vi "AIT 1553 RT Driver VI.vi"(7 "Operation":T1, 11 "Device Reference in":T2 format="%.0x") -> (0 "Error Code":i32)   [LabVIEW 2013, in "AIT 1553 Custom Device.lvlib"]
uses:
  AIT 1553 Custom Device.lvlib
  <vilib>/NI Veristand/Custom Device API/Custom Device Item Ref.ctl
  <vilib>/NI Veristand/Custom Device API/Hardware Interface Driver VI Operation.ctl
  RT Controls/AIT 1553  - RT Data.ctl
  RT Controls/AIT 1553 - RT HW Channel.ctl
  RT Controls/AIT 1553 - Bus Section.ctl
  RT Controls/AIT 1553 - RT Message Settings.ctl
  <vilib>/NI Veristand/Custom Device API/Block Data Reference.ctl
  <vilib>/NI Veristand/Custom Device API/Data Reference.ctl
  RT Controls/AIT 1553 - Driver Data.ctl
  Controls and Global/Start Bit.ctl
  Controls and Global/Number of Bits.ctl
  RT Controls/AIT 1553 - Board Config Info.ctl
  RT Controls/AIT 1553 - Hardware Type.ctl
  RT Controls/Error Qs.ctl
  RT Controls/Status Channels Config.ctl
  RT Controls/FIFO.ctl
  RT Controls/Label Transfer Config.ctl
  <vilib>/NI Veristand/Custom Device Tools/Custom Device Utility Library/RT Debug String Color Spec.ctl
  RT Controls/Async Loop Control Enum.ctl
  RT Controls/ReadWrite Selector.ctl
  SubVIs/Data Ref FGV.vi
  <vilib>/NI Veristand/Custom Device API/NI VeriStand - Set Channel Value by Data Reference.vi
  SubVIs/Error/Push Error if Different.vi
  SubVIs/Error/Print Error.vi
  SubVIs/Init/AIT 1553 - Separate Tx-Rx Messages.vi
  SubVIs/Init/AIT 1553 - Parse RT Channels.vi
  SubVIs/Init/AIT 1553 - Parse BM Channels.vi
  SubVIs/Init/AIT 1553 - Parse BC Channels.vi
  Controls and Global/Global.vi
  SubVIs/Init/AIT 1553 - Get Index and Length.vi
  <vilib>/NI Veristand/Custom Device API/Global Data Refs.vi
  <vilib>/NI Veristand/Custom Device API/Custom Device API.lvlib
  <instrlib>/AIT 1553/AIT 1553.lvlib
  <vilib>/NI Veristand/Custom Device Tools/Custom Device Utility Library/Custom Device Utility Library.lvlib
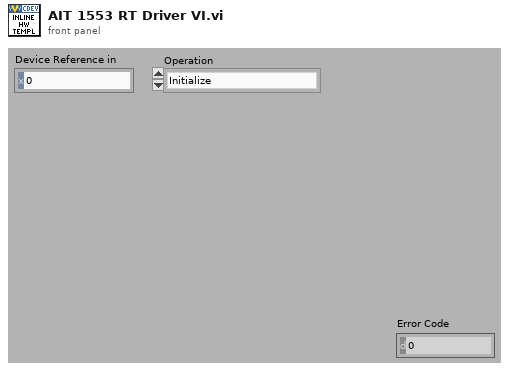
[diagram p1: front panel]
types:
  T1 = typedef "Custom Device API.lvlib/Hardware Interface Driver VI Operation.ctl" = enum16{"Initialize", "Start", "Read Data from HW", "Write Data to HW", "Close"}
  T2 = typedef "Custom Device API.lvlib/Custom Device Item Ref.ctl" = u64
  T3 = typedef "AIT 1553 Custom Device.lvlib/AIT 1553  - RT Data.ctl" = cluster{"HWInput Channels":T4[], "HWOutput Channels":T4[], "Bus Config Info":T12, "Start":refnum<notifier>, "HWIn BaseRate - BC or RT":i64, "HWOut BaseRate - BC or RT":i64, "HWIn BaseRate - BM":i64, "Error Qs":T14, "Error Pub Q":refnum<queue>, "Status Config":T15, "FIFOs":T16, "VI Refs":refnum<vi>[], "Label Transfer Config":T17, "Acyclic Frame Refs":T2[]}
  T4 = typedef "AIT 1553 Custom Device.lvlib/AIT 1553 - RT HW Channel.ctl" = cluster{"channel #":u16, "channel handle":u32, "Bus Section":T5, "Msg Names":string[], "Message Settings":T6[]}
  T5 = typedef "AIT 1553 Custom Device.lvlib/AIT 1553 - Bus Section.ctl" = enum16{"BC", "BM", "RT"}
  T6 = typedef "AIT 1553 Custom Device.lvlib/AIT 1553 - RT Message Settings.ctl" = cluster{"Name":string, "xmlName":string, "Tx-Rx_T-Tx":bool, "RT_Address":u8, "RT_SA_Address":u8, "Block Data Refs":T7[], "Values Array":dbl[], "Length":i32, "Words":i32, "FIFO Index":i32, "RX Word":u32, "transfer handle":u32, "IterationOffset":i32, "Default Msg Data":u16[], "Driver Data":T9, "Status Data":u32[]}
  T7 = typedef "Custom Device API.lvlib/Block Data Reference.ctl" = cluster{"Data Reference":T8, "Offset":i32, "Length":i32}
  T8 = typedef "Custom Device API.lvlib/Data Reference.ctl" = i32
  T9 = typedef "AIT 1553 Custom Device.lvlib/AIT 1553 - Driver Data.ctl" = cluster{"First Word":T10[], "Start Bit":T10[], "Num Bits":T11[], "Decimation":i32, "IterationOffset":i32, "transfer handle":u32, "Signed?":bool[], "ScaleFac":dbl[], "ScaleOffset":dbl[]}
  T10 = typedef "AIT 1553 Custom Device.lvlib/Start Bit.ctl" = i32
  T11 = typedef "AIT 1553 Custom Device.lvlib/Number of Bits.ctl" = i32
  T12 = typedef "AIT 1553 Custom Device.lvlib/AIT 1553 - Board Config Info.ctl" = cluster{"board handle":u32, "channel  handle":u32, "bus controller handle":u32, "bus monitor handle":u32, "remote terminal handle array":u32[], "1553 Hardware Type":T13, "Monitor Data Handle":u32}
  T13 = typedef "AIT 1553 Custom Device.lvlib/AIT 1553 - Hardware Type.ctl" = enum16{"AIM board", "AIT Board"}
  T14 = typedef "AIT 1553 Custom Device.lvlib/Error Qs.ctl" = cluster{"BC HWin":refnum<queue>, "BM HWin":refnum<queue>, "RT HWin":refnum<queue>, "BC HWOut":refnum<queue>, "RT HWOut":refnum<queue>}
  T15 = typedef "AIT 1553 Custom Device.lvlib/Status Channels Config.ctl" = cluster{"Error Data Ref":T8, "HWIn Count Ref":T8, "HWIn Count Idx":i32, "HWOut Count Ref":T8, "HWOut Count Idx":i32, "HWIn Dur Ref":T8, "HWIn Dur Idx":i32, "HWOut Dur Ref":T8, "HWOut Dur Idx":i32}
  T16 = typedef "AIT 1553 Custom Device.lvlib/FIFO.ctl" = cluster{"HWIn FIFOs":refnum<k33>[], "HWOut FIFOs":refnum<k33>[], "HWIn Buf":dbl[], "HWOut Buf":dbl[], "Empty HWIn FIFOs":bool[], "HWIn Buf Indices":i32[], "HWOut Buf Indices":i32[], "HWIn Buf Lengths":i32[], "HWOut Buf Lengths":i32[]}
  T17 = typedef "AIT 1553 Custom Device.lvlib/Label Transfer Config.ctl" = cluster{"Block Data Refs":T7[], "Values Array":dbl[]}
  T18 = typedef "AIT 1553 Custom Device.lvlib/Async Loop Control Enum.ctl" = enum16{"Launch", "Start", "Stop"}
  T19 = typedef "AIT 1553 Custom Device.lvlib/ReadWrite Selector.ctl" = enum16{"Inline Read", "Inline Write", "Async HWIn", "Async HWOut"}
  T20 = typedef "Custom Device Utility Library.lvlib/RT Debug String Color Spec.ctl" = u16
  T21 = typedef "AIT 1553 Custom Device.lvlib/FIFO Idx Qs.ctl" = cluster{"HWInput Q":refnum<queue>, "HWOutput Q":refnum<queue>}
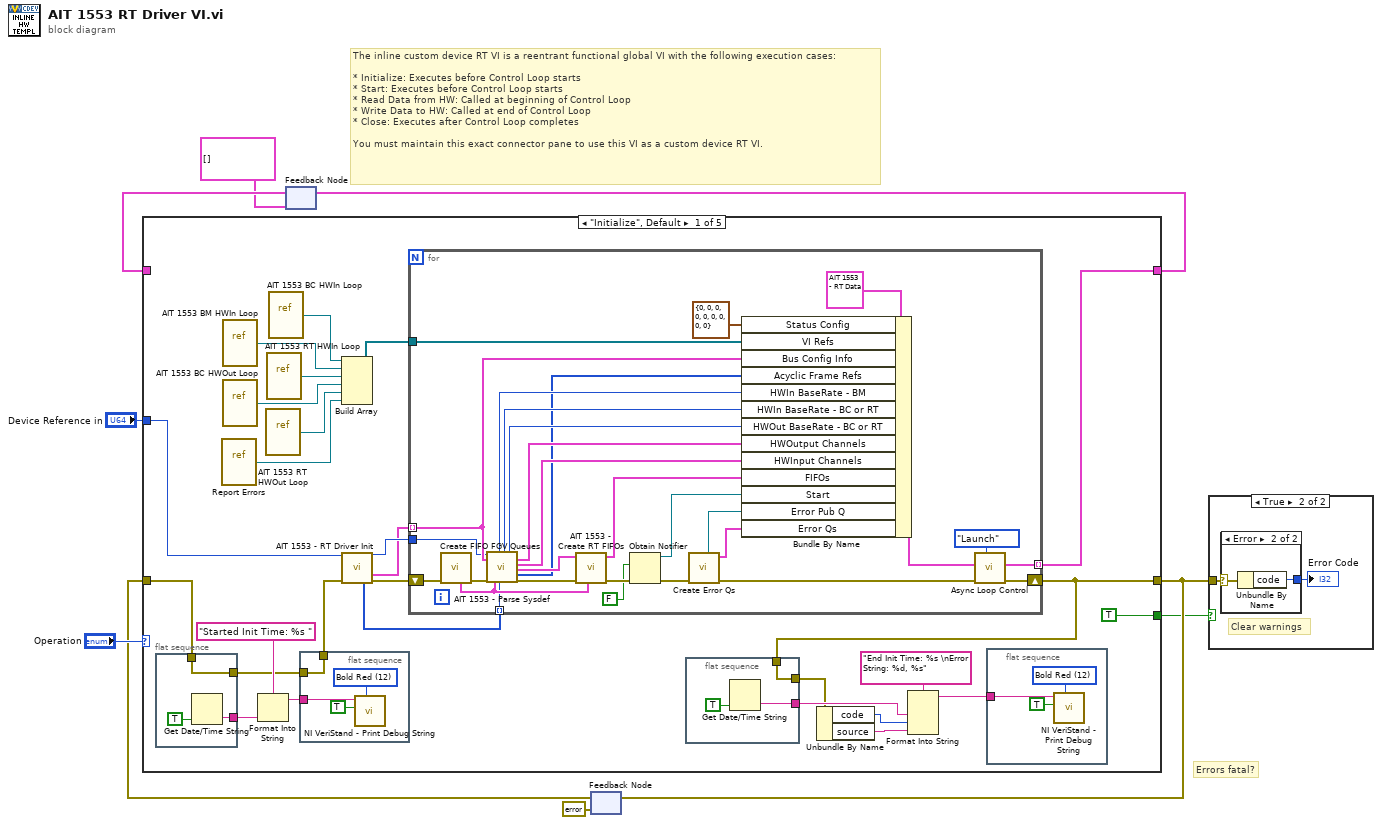
[diagram p0: block diagram]
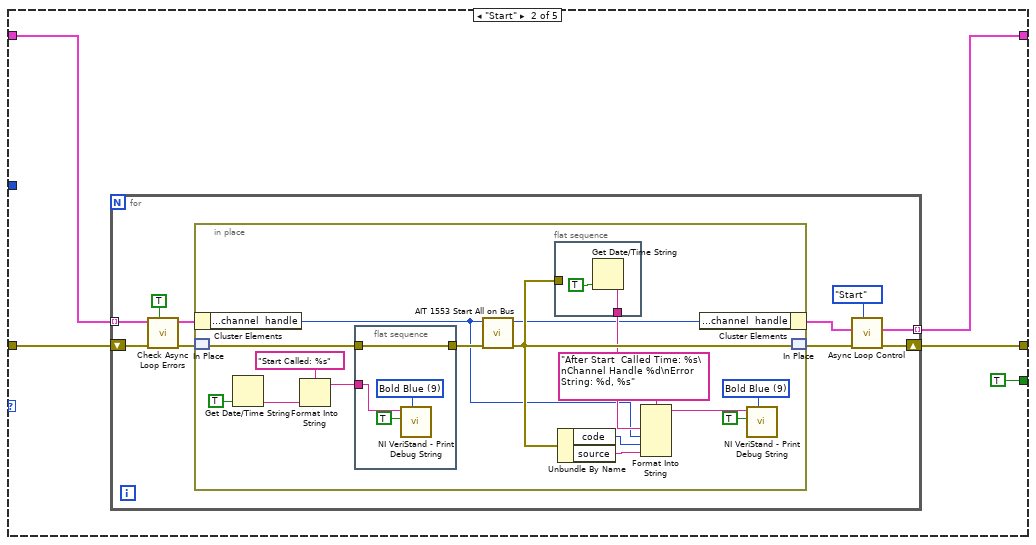
[diagram p4: hidden frame]
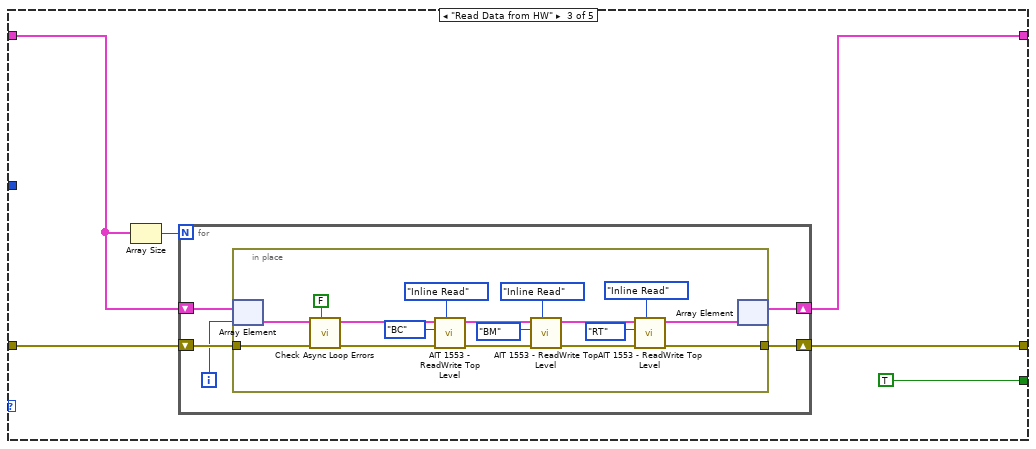
[diagram p5: hidden frame]
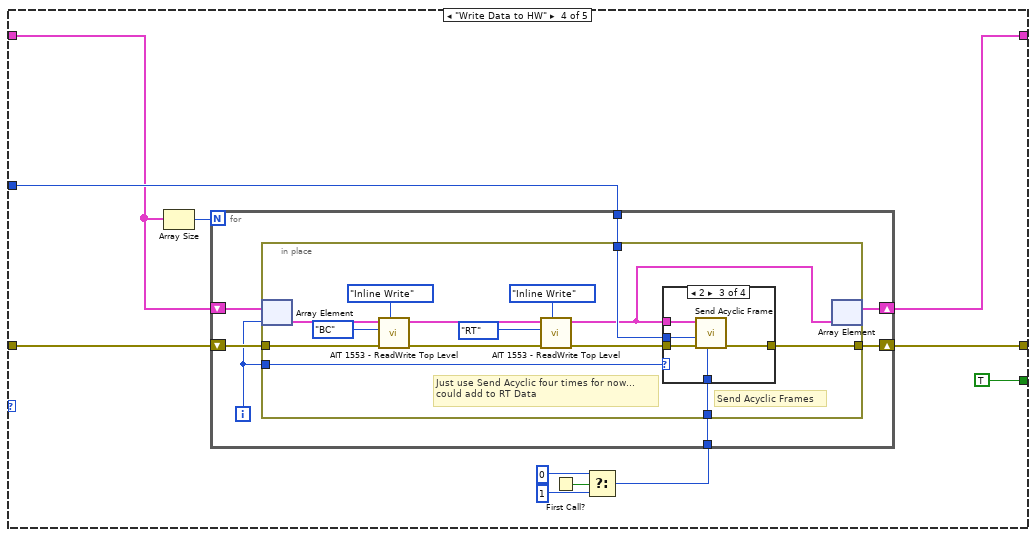
[diagram p6: hidden frame]
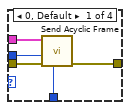
[diagram p7: hidden frame]
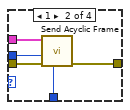
[diagram p8: hidden frame]
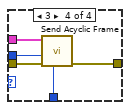
[diagram p9: hidden frame]
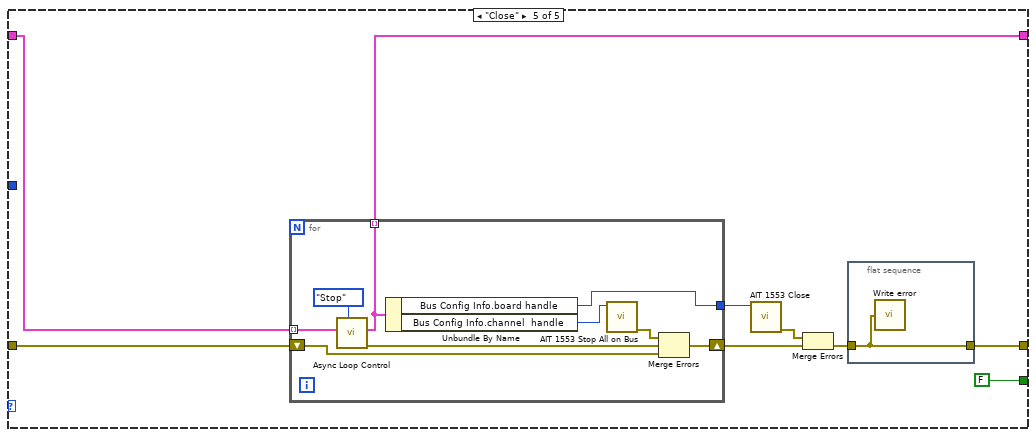
[diagram p10: hidden frame]
diagram:
  # "Errors fatal?"
  # "The inline custom device RT VI is a reentrant functional global VI with the following execution cases:\n\n* Initialize: Executes before Control Loop starts\n* Start: Executes before Control Loop starts\n* Read Data from HW: Called at beginning of Control Loop\n* Write Data to HW: Called at end of Control Loop\n* Close: Executes after Control Loop completes\n\nYou must maintain this exact connector pane to use this VI as a custom device RT VI."
  n1 = feedback #1(T3[] []) -> (w3:T3[])
  n2 = feedback #2(errorcluster {"status"=FALSE, "code"=0, "source"=""} ("error out")) -> (w6:errorcluster)
  n3 = case shown="\"Initialize\", Default" "Operation" {
    tunnel: w3 -> [_ w80 w117 w149 w202]
    tunnel: "Device Reference in" -> [w16 _ _ w151 _]
    tunnel: [w11 w79 w116 w148 w201] -> w2
    tunnel: [w12 w83 w119 w152 w200] -> w7
    tunnel: w6 -> [w17 w82 w121 w154 w204]
    tunnel: [TRUE TRUE TRUE TRUE FALSE] -> w5
    frame "Initialize", Default {
      n4 = flat-sequence {
        tunnel: [w68] -> w28
        tunnel: w17 -> [w66]
        tunnel: [w66] -> w27
        frame #0 {
          n5 = Get Date/Time String(want seconds? (F)=TRUE) -> (time string=w68:string)  [unwired: 2 in, 1 out]
        }
      }
      n6 = vi-ref "Report Errors.vi"() -> (w19:refnum<vi>)
      n7 = vi-ref "AIT 1553 BM HWIn Loop.vi"() -> (w23:refnum<vi>)
      n8 = vi-ref "AIT 1553 BC HWOut Loop.vi"() -> (w21:refnum<vi>)
      n9 = Format Into String(format string="Started Init Time: %s ", w28) -> (resulting string=w29:string)  [unwired: 2 in, 1 out]
      n10 = vi-ref "AIT 1553 RT HWOut Loop.vi"() -> (w20:refnum<vi>)
      n11 = vi-ref "AIT 1553 RT HWIn Loop.vi"() -> (w22:refnum<vi>)
      n12 = vi-ref "AIT 1553 BC HWIn Loop.vi"() -> (w24:refnum<vi>)
      n13 = flat-sequence {
        tunnel: w29 -> [w71]
        tunnel: w27 -> [w72]
        tunnel: [w72] -> w26
        frame #0 {
          w70 = T20 12 items=["Plain White"=7, "Bold White"=15, "Bold Blue"=9, "Bold Green"=10, "Bold Red"=12] ("Attribute")
          n14 = call <vilib>:"NI VeriStand - Print Debug String.vi"("Attribute"=w70, "Add to log file? (T)"=TRUE, "Message"=w71) -> ()  [unwired: 8 in, 1 out]
        }
      }
      n15 = Build Array(w24, w23, w22, w21, w20, w19) -> (w18:refnum<vi>[])
      n16 = call "AIT 1553 - RT Driver Init.vi"("Device Reference in"=w16, "error in"=w26) -> ("Device Reference out"=w14:T2, "Bus Config Info Array"=w13:T12[], "Child Refs - 1553 Busses"=w10:T2[], "error out"=w15:errorcluster)  [unwired: 8 in, 2 out]
      n17 = for {
        tunnel: w18 -> [w49]
        tunnel: w13 -> [w48] mode=indexing
        tunnel: w14 -> [w44]
        shift-right: [w41] -> w12
        shift-left: w15 -> [w47]
        tunnel: [w39] -> w11 mode=indexing
        tunnel: w10 -> [w37] mode=indexing
        n18 = call "Create FIFO FGV Queues.vi"("error in (no error)"=w47) -> ("error out"=w46:errorcluster, "BC FIFO Idx Qs"=w45:T21)  [unwired: 9 in]
        n19 = call "AIT 1553 - Parse Sysdef.vi"("Device Reference in"=w44, "Bus Config Info"=w48, "error in (no error)"=w46, "FIFO Idx Qs"=w45, "Bus Page Ref"=w37) -> ("HWIn BaseRate BM"=w52:i32, "HWIn BaseRate"=w58:i32, "HWOut BaseRate"=w59:i32, "HWOutput Section Data"=w57:T4[], "HWInput Section Data"=w54:T4[], "output cluster"=w53:T16, "Bus Controller Page Acyclic Frame Refs out"=w50:T2[], "error out"=w65:errorcluster)  [unwired: 6 in, 1 out]
        n20 = call "AIT 1553 - Create RT FIFOs.vi"("FIFO Idx Qs"=w45, "error in (no error)"=w65, "input cluster"=w53) -> ("error out"=w64:errorcluster, "output cluster"=w60:T16)  [unwired: 7 in]
        n21 = Obtain Notifier(notification data type=FALSE, error in (no error)=w64) -> (notifier out=w56:refnum<notifier>, error out=w62:errorcluster)  [unwired: 2 in, 1 out]
        n22 = call "Create Error Qs.vi"("error in (no error)"=w62) -> ("error out"=w42:errorcluster, "Error Qs"=w55:T14, "Error Publishing Q"=w61:refnum<queue>)  [unwired: 8 in]
        n23 = Bundle By Name(cluster=T3 {"HWInput Channels"=[], "HWOutput Channels"=[], "Bus Config Info"={"board handle"=0, "channel  handle"=0, "bus controller handle"=0, "bus monitor handle"=0, "remote terminal handle array"=[], "1553 Hardware Type"=enum."AIM board", "Monitor Data Handle"=0}, "Start"=refnum, "HWIn BaseRate - BC or RT"=0, "HWOut BaseRate - BC or RT"=0, "HWIn BaseRate - BM"=0, "Error Qs"={"BC HWin"=refnum, "BM HWin"=refnum, "RT HWin"=refnum, "BC HWOut"=refnum, "RT HWOut"=refnum}, "Error Pub Q"=refnum, "Status Config"={"Error Data Ref"=0, "HWIn Count Ref"=0, "HWIn Count Idx"=0, "HWOut Count Ref"=0, "HWOut Count Idx"=0, "HWIn Dur Ref"=0, "HWIn Dur Idx"=0, "HWOut Dur Ref"=0, "HWOut Dur Idx"=0}, "FIFOs"={"HWIn FIFOs"=[], "HWOut FIFOs"=[], "HWIn Buf"=[], "HWOut Buf"=[], "Empty HWIn FIFOs"=[], "HWIn Buf Indices"=[], "HWOut Buf Indices"=[], "HWIn Buf Lengths"=[], "HWOut Buf Lengths"=[]}, "VI Refs"=[], "Label Transfer Config"={"Block Data Refs"=[], "Values Array"=[]}, "Acyclic Frame Refs"=[]} ("RT Data"), "Status Config"=T15 {"Error Data Ref"=0, "HWIn Count Ref"=0, "HWIn Count Idx"=0, "HWOut Count Ref"=0, "HWOut Count Idx"=0, "HWIn Dur Ref"=0, "HWIn Dur Idx"=0, "HWOut Dur Ref"=0, "HWOut Dur Idx"=0}, "VI Refs"=w49, "Bus Config Info"=w48, "Acyclic Frame Refs"=w50, "HWIn BaseRate - BM"=w52, "HWIn BaseRate - BC or RT"=w58, "HWOut BaseRate - BC or RT"=w59, "HWOutput Channels"=w57, "HWInput Channels"=w54, "FIFOs"=w60, "Start"=w56, "Error Pub Q"=w61, "Error Qs"=w55) -> (w40:T3)
        n24 = call "Async Loop Control.vi"("Action"=Async_Loop_Control_Enum."Launch", "error in (no error)"=w42, "RT Data In"=w40) -> ("error out"=w41:errorcluster, "RT Data Out"=w39:T3)  [unwired: 7 in]
      }
      n25 = flat-sequence {
        tunnel: [w75] -> w32
        tunnel: w12 -> [w73]
        tunnel: [w73] -> w25
        frame #0 {
          n26 = Get Date/Time String(want seconds? (F)=TRUE) -> (time string=w75:string)  [unwired: 2 in, 1 out]
        }
      }
      n27 = Unbundle By Name(w25) -> ("code"=w31:i32, "source"=w34:string)
      n28 = Format Into String(format string="End Init Time: %s \nError String: %d, %s", w32, w31, w34) -> (resulting string=w35:string)  [unwired: 2 in, 1 out]
      n29 = flat-sequence {
        tunnel: w35 -> [w76]
        frame #0 {
          w78 = T20 12 items=["Plain White"=7, "Bold White"=15, "Bold Blue"=9, "Bold Green"=10, "Bold Red"=12] ("Attribute")
          n30 = call <vilib>:"NI VeriStand - Print Debug String.vi"("Attribute"=w78, "Add to log file? (T)"=TRUE, "Message"=w76) -> ()  [unwired: 8 in, 1 out]
        }
      }
    }
    frame "Start" {
      n31 = for {
        tunnel: w80 -> [w87] mode=indexing
        tunnel: [w85] -> w79 mode=indexing
        shift-right: [w92] -> w83
        shift-left: w82 -> [w91]
        n32 = call "Check Async Loop Errors.vi"("Init"=TRUE, "error in (no error)"=w91, "RT Data in"=w87) -> ("error out"=w90:errorcluster, "RT Data Out"=w89:T3)  [unwired: 7 in]
        n33 = in-place {
          w99 = T20 9 items=["Plain White"=7, "Bold White"=15, "Bold Blue"=9, "Bold Green"=10, "Bold Red"=12] ("Attribute")
          n34 = in-place-cluster #3(w89) -> ("Bus Config Info.channel  handle"=w96:u32)
          n35 = in-place-match #4(w90) -> (w106:errorcluster)
          n36 = Get Date/Time String(want seconds? (F)=TRUE) -> (time string=w105:string)  [unwired: 2 in, 1 out]
          n37 = Format Into String(format string="Start Called: %s", w105) -> (resulting string=w104:string)  [unwired: 2 in, 1 out]
          n38 = flat-sequence {
            tunnel: w104 -> [w112]
            tunnel: w106 -> [w115]
            tunnel: [w115] -> w103
            frame #0 {
              w114 = T20 9 items=["Plain White"=7, "Bold White"=15, "Bold Blue"=9, "Bold Green"=10, "Bold Red"=12] ("Attribute")
              n39 = call <vilib>:"NI VeriStand - Print Debug String.vi"("Attribute"=w114, "Add to log file? (T)"=TRUE, "Message"=w112) -> ()  [unwired: 8 in, 1 out]
            }
          }
          n40 = call <instrlib>:"AIT 1553 Start All on Bus.vi"("error in"=w103, "channel handle in"=w96) -> ("error out"=w102:errorcluster, "channel handle out"=w94:u32)  [unwired: 8 in]
          n41 = flat-sequence {
            tunnel: w102 -> [_]
            tunnel: [w111] -> w101
            frame #0 {
              n42 = Get Date/Time String(want seconds? (F)=TRUE) -> (time string=w111:string)  [unwired: 2 in, 1 out]
            }
          }
          n43 = Unbundle By Name(w102) -> ("code"=w107:i32, "source"=w109:string)
          n44 = Format Into String(format string="After Start  Called Time: %s\nChannel Handle %d\nError String: %d, %s", w101, w96, w107, w109) -> (resulting string=w97:string)  [unwired: 2 in, 1 out]
          n45 = in-place-cluster #3("Bus Config Info.channel  handle"=w94) -> (w86:T3)
          n46 = call <vilib>:"NI VeriStand - Print Debug String.vi"("Attribute"=w99, "Add to log file? (T)"=TRUE, "Message"=w97) -> ()  [unwired: 8 in, 1 out]
          n47 = in-place-match #4(w102) -> (w88:errorcluster)
        }
        n48 = call "Async Loop Control.vi"("Action"=Async_Loop_Control_Enum."Start", "error in (no error)"=w88, "RT Data In"=w86) -> ("error out"=w92:errorcluster, "RT Data Out"=w85:T3)  [unwired: 7 in]
      }
    }
    frame "Read Data from HW" {
      n49 = Array Size(array=w117) -> (size(s)=w118:i32)
      n50 = for {
        N: w118 -> [_]
        shift-right: [w125] -> w119
        shift-left: w121 -> [w126]
        shift-right: [w122] -> w116
        shift-left: w117 -> [w124]
        i -> [w123]
        n51 = in-place {
          in-place-border: w126 -> [w141]
          in-place-border: [w133] -> w125
          n52 = in-place-array #5(w124, w123) -> (w129:T3)
          n53 = call "Check Async Loop Errors.vi"("Init"=FALSE, "error in (no error)"=w141, "RT Data in"=w129) -> ("error out"=w142:errorcluster, "RT Data Out"=w143:T3)  [unwired: 7 in]
          n54 = call "AIT 1553 - ReadWrite Top Level.vi"("Mode"=ReadWrite_Selector."Inline Read", "error in (no error)"=w142, "Bus Section"=AIT_1553_-_Bus_Section."BC", "RT Data in"=w143) -> ("error out"=w137:errorcluster, "RT Data out"=w135:T3)  [unwired: 6 in]
          n55 = call "AIT 1553 - ReadWrite Top Level.vi"("Mode"=ReadWrite_Selector."Inline Read", "error in (no error)"=w137, "Bus Section"=AIT_1553_-_Bus_Section."BM", "RT Data in"=w135) -> ("error out"=w136:errorcluster, "RT Data out"=w134:T3)  [unwired: 6 in]
          n56 = call "AIT 1553 - ReadWrite Top Level.vi"("Mode"=ReadWrite_Selector."Inline Read", "error in (no error)"=w136, "Bus Section"=AIT_1553_-_Bus_Section."RT", "RT Data in"=w134) -> ("error out"=w133:errorcluster, "RT Data out"=w128:T3)  [unwired: 6 in]
          n57 = in-place-array #5(w128) -> (w122:T3[])  [unwired: 1 out]
        }
      }
    }
    frame "Write Data to HW" {
      n58 = Array Size(array=w149) -> (size(s)=w150:i32)
      n59 = First Call?() -> (First Call?: T/F=w145:bool)
      n60 = Select(t=0 ("Index"), s=w145, f=1 ("Index")) -> (s? t:f=w144:i32)
      n61 = for {
        N: w150 -> [_]
        tunnel: w151 -> [w159]
        shift-right: [w157] -> w148
        shift-left: w149 -> [w158]
        shift-right: [w160] -> w152
        shift-left: w154 -> [w161]
        tunnel: w144 -> [w156]
        i -> [w155]
        n62 = in-place {
          in-place-border: w161 -> [w175]
          in-place-border: [w167] -> w160
          in-place-border: w159 -> [w166]
          in-place-border: w156 -> [w163]
          in-place-border: w155 -> [w162]
          # "Just use Send Acyclic four times for now...\ncould add to RT Data"
          # "Send Acyclic Frames"
          n63 = in-place-array #6(w158, w155) -> (w165:T3)
          n64 = call "AIT 1553 - ReadWrite Top Level.vi"("Mode"=ReadWrite_Selector."Inline Write", "error in (no error)"=w175, "Bus Section"=AIT_1553_-_Bus_Section."BC", "RT Data in"=w165) -> ("error out"=w171:errorcluster, "RT Data out"=w172:T3)  [unwired: 6 in]
          n65 = call "AIT 1553 - ReadWrite Top Level.vi"("Mode"=ReadWrite_Selector."Inline Write", "error in (no error)"=w171, "Bus Section"=AIT_1553_-_Bus_Section."RT", "RT Data in"=w172) -> ("error out"=w168:errorcluster, "RT Data out"=w164:T3)  [unwired: 6 in]
          n66 = case shown="2" w162 {
            tunnel: w168 -> [w180 w185 w190 w195]
            tunnel: [w179 w184 w189 w194] -> w167
            tunnel: w166 -> [w178 w183 w188 w193]
            tunnel: w164 -> [w177 w182 w187 w192]
            tunnel: w163 -> [w176 w181 w186 w191]
            frame 0, Default {
              n67 = call "Send Acyclic Frame.vi"("Index"=w176, "error in (no error)"=w180, "Device Reference in"=w178, "RT Data out"=w177) -> ("error out"=w179:errorcluster)  [unwired: 7 in]
            }
            frame 1 {
              n68 = call "Send Acyclic Frame.vi"("Index"=w181, "error in (no error)"=w185, "Device Reference in"=w183, "RT Data out"=w182) -> ("error out"=w184:errorcluster)  [unwired: 7 in]
            }
            frame 2 {
              n69 = call "Send Acyclic Frame.vi"("Index"=w186, "error in (no error)"=w190, "Device Reference in"=w188, "RT Data out"=w187) -> ("error out"=w189:errorcluster)  [unwired: 7 in]
            }
            frame 3 {
              n70 = call "Send Acyclic Frame.vi"("Index"=w191, "error in (no error)"=w195, "Device Reference in"=w193, "RT Data out"=w192) -> ("error out"=w194:errorcluster)  [unwired: 7 in]
            }
          }
          n71 = in-place-array #6(w164) -> (w157:T3[])  [unwired: 1 out]
        }
      }
    }
    frame "Close" {
      n72 = for {
        tunnel: w202 -> [w212] mode=indexing
        tunnel: [w211] -> w201 mode=indexing
        shift-right: [w207] -> w198
        shift-left: w204 -> [w209]
        tunnel: [w208] -> w199
        n73 = call "Async Loop Control.vi"("Action"=Async_Loop_Control_Enum."Stop", "RT Data In"=w212) -> ("error out"=w214:errorcluster, "RT Data Out"=w211:T3)  [unwired: 8 in]
        n74 = Unbundle By Name(w211) -> ("Bus Config Info.board handle"=w208:u32, "Bus Config Info.channel  handle"=w210:u32)
        n75 = call <instrlib>:"AIT 1553 Stop All on Bus.vi"("channel handle in"=w210) -> ("error out"=w206:errorcluster)  [unwired: 9 in, 1 out]
        n76 = Merge Errors(w206, w214, w209) -> (w207:errorcluster)
      }
      n77 = call <instrlib>:"AIT 1553 Close.vi"("board handle in"=w199) -> ("error out"=w196:errorcluster)  [unwired: 10 in]
      n78 = Merge Errors(w196, w198) -> (w197:errorcluster)
      n79 = flat-sequence {
        tunnel: w197 -> [w205]
        tunnel: [w205] -> w200
        frame #0 {
          n80 = call "Write error.vi"("error in (no error)"=w205) -> ()
        }
      }
    }
  }
  n81 = feedback-in #1(w2) -> ()
  n82 = feedback-in #2(w7) -> ()
  n83 = case shown="True" w5 {
    tunnel: w7 -> [_ w215]
    frame False {
    }
    frame True {
      # "Clear warnings"
      n84 = case shown="Error" w215 {
        selector: w215 -> [_ w218]
        tunnel: [_ w217] -> w216
        frame No Error {
        }
        frame Error {
          n85 = Unbundle By Name(w218) -> ("code"=w217:i32)
        }
      }
      "Error Code" <- w216
    }
  }
